vi "Modify OpenG VIs.vi"() -> ()   [LabVIEW 2013]
uses:
  ReentrancyType--Enum.ctl
  ReentrancySettings--Cluster.ctl
panel:
  in  "Path":path
  in  "Exceptions":T1[](array[typedef])=[{"VI Name"="Size of Data from TD", "Reentrancy Type"=enum."Shared Clones Reentrant", "Inline"=FALSE}, {"VI Name"="Get Default Data from TD", "Reentrancy Type"=enum."Shared Clones Reentrant", "Inline"=FALSE}]
  in  "Reentrancy Type":T2=enum."Preallocate Reentrant"
  in  "Inline":bool=TRUE
  in  "Automatic Error Handling":bool
  in  "Debugging":bool
  # "Settings"
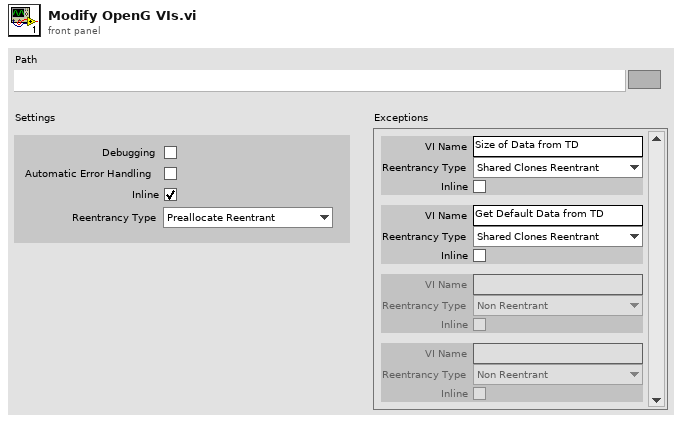
[diagram p1: front panel]
types:
  T1 = typedef "ReentrancySettings--Cluster.ctl" = cluster{"VI Name":string, "Reentrancy Type":T2, "Inline":bool}
  T2 = typedef "ReentrancyType--Enum.ctl" = enum16{"Non Reentrant", "Shared Clones Reentrant", "Preallocate Reentrant"}
  T3 = enum16{"Share clones between instances", "Preallocate clone for each instance"}
  T4 = enum32{"invalid VI type", "Standard VI", "Control VI", "Global VI", "Polymorphic VI", "Configuration VI", "SubSystem", "Facade VI", "Method VI", "Statechart Diagram VI"}
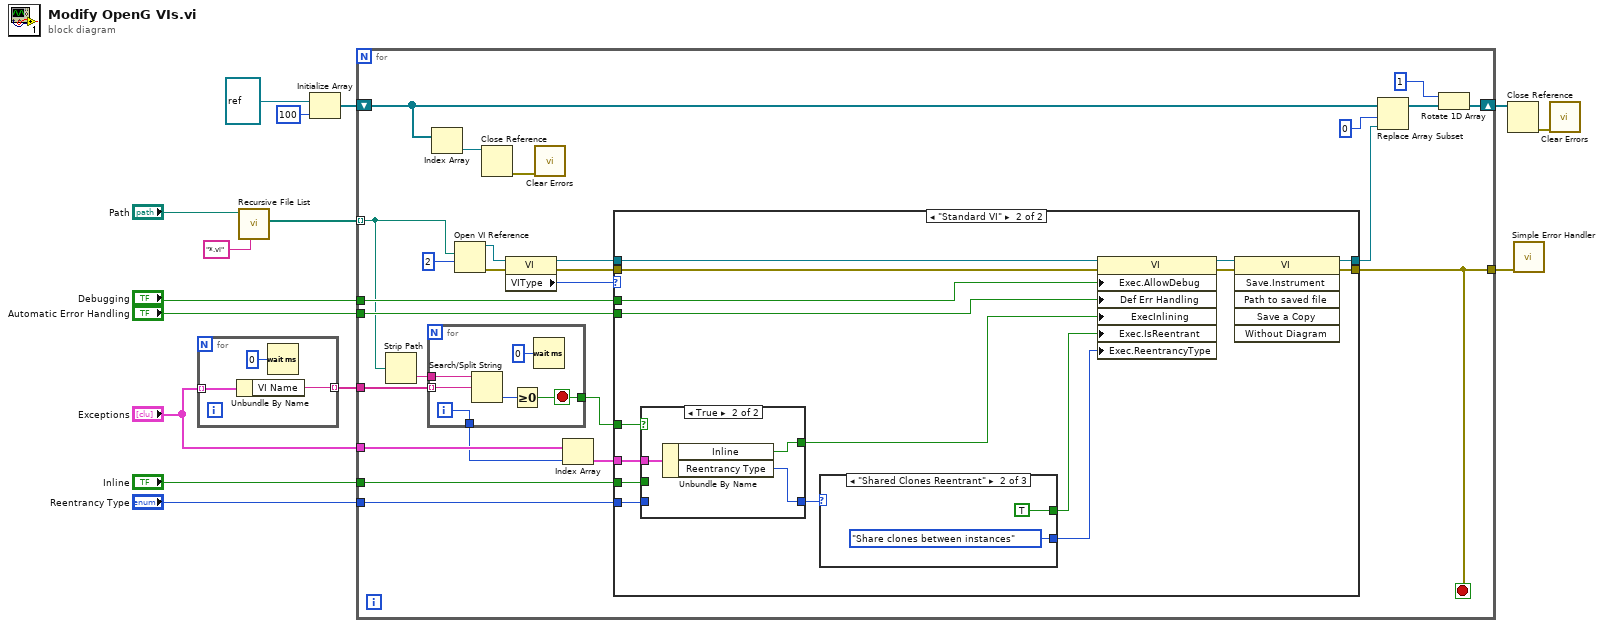
[diagram p0: block diagram]
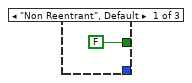
[diagram p4: hidden frame]
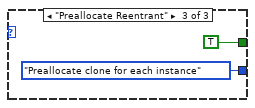
[diagram p5: hidden frame]
diagram:
  n1 = for {
    tunnel: "Exceptions" -> [w18] mode=indexing
    tunnel: [w16] -> w14 mode=indexing
    n2 = Unbundle By Name(w18) -> ("VI Name"=w16:string)
    n3 = Wait (ms)(milliseconds to wait=u32 0) -> ()  [unwired: 1 out]
  }
  n4 = call <vilib>:"Recursive File List.vi"("pattern"="*.vi", "Folder Path"="Path") -> ("All Files in Dir"=w9:path[])  [unwired: 5 in, 4 out]
  n5 = Initialize Array(refnum<vi> refnum ("vi reference"), 100 ("dimension size")) -> (w11:refnum<vi>[])
  n6 = for {
    tunnel: w9 -> [w39] mode=indexing
    tunnel: "Debugging" -> [w43]
    tunnel: "Automatic Error Handling" -> [w42]
    tunnel: "Exceptions" -> [w41]
    tunnel: w14 -> [w38]
    shift-right: [w33] -> w2
    shift-left: w11 -> [w31]
    tunnel: [w20] -> w10
    tunnel: "Reentrancy Type" -> [w23]
    tunnel: "Inline" -> [w22]
    stop <- w20 stop-if-true
    n7 = Strip Path(path=w39) -> (name=w37:string)  [unwired: 1 out]
    n8 = for {
      tunnel: w38 -> [w76] mode=indexing
      tunnel: w37 -> [w77]
      tunnel: [w74] -> w36
      tunnel: [w73] -> w21
      i -> [w74]
      stop <- w73 stop-if-true
      n9 = Search/Split String(string=w77, search string/char (-)=w76) -> (offset of match=w78:i32)  [unwired: 1 in, 2 out]
      n10 = Greater Or Equal To 0?(x=w78) -> (x >= 0?=w73:bool)
      n11 = Wait (ms)(milliseconds to wait=u32 0) -> ()  [unwired: 1 out]
    }
    n12 = Index Array(array=w31) -> (element=w30:refnum<vi>)  [unwired: 1 in]
    n13 = Open VI Reference(vi path=w39, options=2) -> (vi reference=w26:refnum<vi>, error out=w44:errorcluster)  [unwired: 4 in]
    n14 = Close Reference(reference=w30) -> (error out=w29:errorcluster)  [unwired: 1 in]
    n15 = property class="VI"(reference=w26, error in=w44) -> (reference out=w25:refnum<vi>, error out=w27:errorcluster, "VIType"=w24:T4)
    n16 = call <vilib>:"Clear Errors.vi"("error in (no error)"=w29) -> ()  [unwired: 6 in, 1 out]
    n17 = Index Array(array=w41, index=w36) -> (element=w40:T1)
    n18 = case shown="\"Standard VI\"" w24 {
      tunnel: w43 -> [_ w48]
      tunnel: w42 -> [_ w47]
      tunnel: w40 -> [_ w60]
      tunnel: [w45 w59] -> w19
      tunnel: [w46 w58] -> w20
      tunnel: w27 -> [w46 w57]
      tunnel: w25 -> [w45 w56]
      tunnel: w23 -> [_ w55]
      tunnel: w22 -> [_ w54]
      tunnel: w21 -> [_ w51]
      frame Default {
      }
      frame "Standard VI" {
        n19 = case shown="True" w51 {
          tunnel: w60 -> [_ w67]
          tunnel: [w64 w65] -> w50
          tunnel: [w63 w66] -> w49
          tunnel: w54 -> [w64 _]
          tunnel: w55 -> [w63 _]
          frame False {
          }
          frame True {
            n20 = Unbundle By Name(w67) -> ("Inline"=w65:bool, "Reentrancy Type"=w66:T2)
          }
        }
        n21 = case shown="\"Shared Clones Reentrant\"" w49 {
          tunnel: [_ T3."Share clones between instances" ("Execution:Reentrancy Type") T3."Preallocate clone for each instance" ("Execution:Reentrancy Type")] -> w53
          tunnel: [FALSE TRUE TRUE] -> w52
          frame "Non Reentrant", Default {
          }
          frame "Shared Clones Reentrant" {
          }
          frame "Preallocate Reentrant" {
          }
        }
        n22 = property class="VI"(reference=w56, error in=w57, "Exec.AllowDebug"=w48, "Def Err Handling"=w47, "ExecInlining"=w50, "Exec.IsReentrant"=w52, "Exec.ReentrancyType"=w53) -> (reference out=w61:refnum<vi>, error out=w62:errorcluster)
        n23 = invoke class="VI" method="Save.Instrument"(reference=w61, error in=w62) -> (reference out=w59:refnum<vi>, error out=w58:errorcluster)  [unwired: 4 in, 4 out]
      }
    }
    n24 = Replace Array Subset(array=w31, new element=w19, index=0) -> (w35:refnum<vi>[])
    n25 = Rotate 1D Array(1:w35, 2:1 ("n")) -> (0:w33:refnum<vi>[])
  }
  n26 = Close Reference(reference=w2) -> (error out=w1:errorcluster)  [unwired: 1 in]
  n27 = call <vilib>:"Simple Error Handler.vi"("error in (no error)"=w10) -> ()  [unwired: 4 in, 5 out]
  n28 = call <vilib>:"Clear Errors.vi"("error in (no error)"=w1) -> ()  [unwired: 6 in, 1 out]
